vi "Run.vi"(8 "error in (no error)":errorcluster caption="entrée d'erreur (pas d'erreur)", 9 "y_score":string[][](array[string]), 10 "y_true":string[][](array[string]), 11 "Roc_Curve.lvclass":refnum<class "Roc_Curve.lvclass">) -> (0 "error out":errorcluster caption="sortie d'erreur", 2 "Data":T1, 3 "Roc_Curve.lvclass":refnum<class "Roc_Curve.lvclass">)   [LabVIEW 2020, in "Roc_Curve.lvclass"]
doc: "Returns :\n\n- fpr : array, shape = [>2]\nIncreasing false positive rates such that element i is the false positive rate of predictions with score >= thresholds[i].\n\n- tpr : array, shape = [>2]\nIncreasing true positive rates such that element i is the true positive rate of predictions with score >= thresholds[i].\n\n- thresholds : array, shape = [n_thresholds]\nDecreasing thresholds on the decision function used to compute fpr and tpr. thresholds[0] represents no instances being predicted and is arbitrarily set to max(y_score) + 1."
uses:
  Roc_Curve.lvclass
  Roc_Curve.lvclass/Roc_Curve.ctl
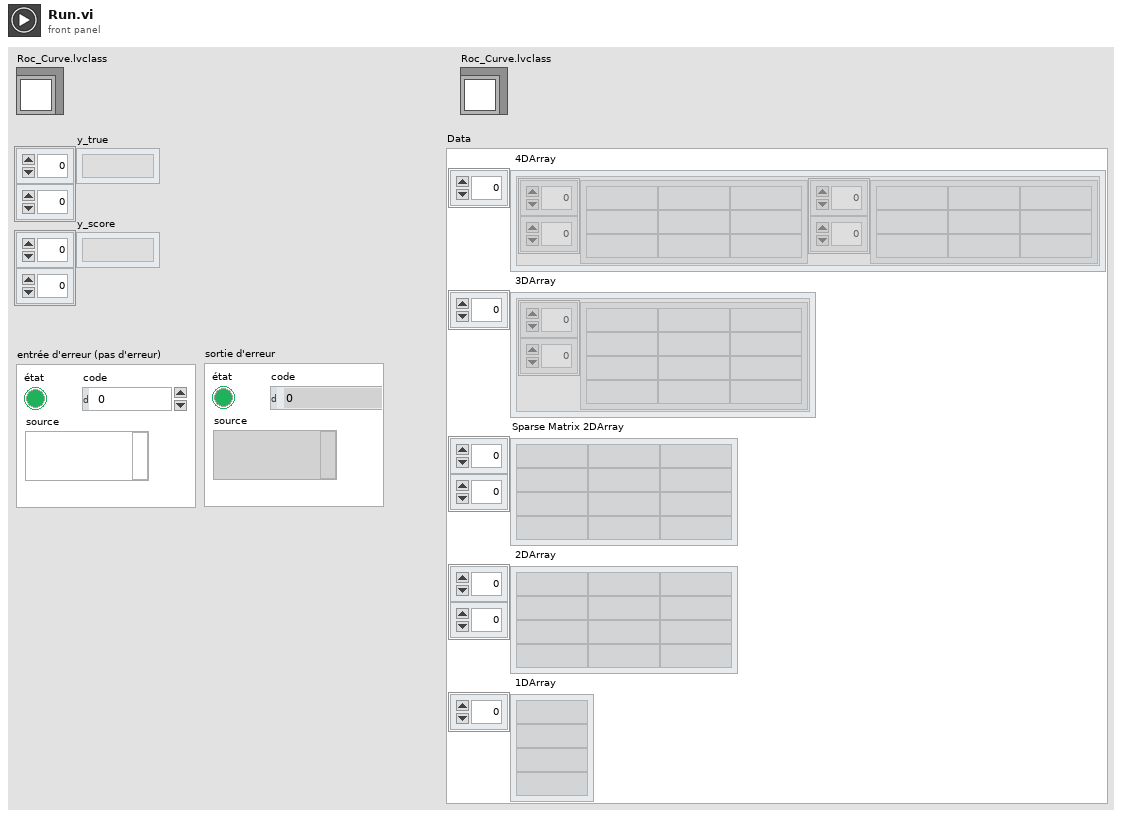
[diagram p1: front panel]
types:
  T1 = cluster{" 4DArray":cluster{"1":string[][], "2":string[][]}[], " 3DArray":cluster{"Tableau":string[][]}[], "Sparse Matrix 2DArray":string[][], " 2DArray":string[][], " 1DArray":string[]}
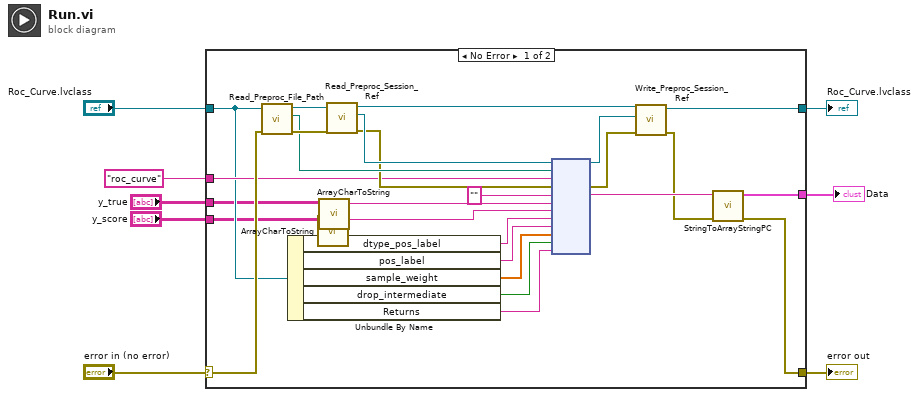
[diagram p0: block diagram]
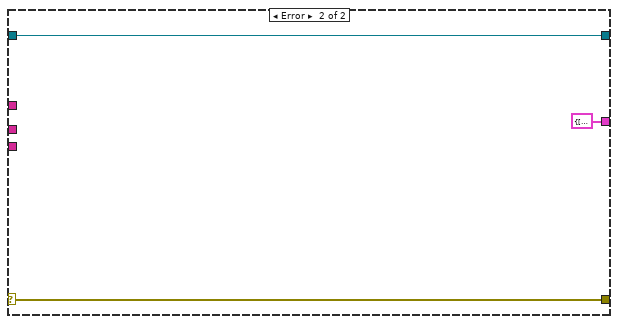
[diagram p2: hidden frame]
diagram:
  n1 = case shown="No Error" "error in (no error)" {
    selector: "error in (no error)" -> [w25 w37]
    tunnel: [w10 w37] -> w7
    tunnel: [w13 w36] -> w5
    tunnel: "Roc_Curve.lvclass" -> [w23 w36]
    tunnel: "roc_curve" -> [w24 _]
    tunnel: "y_true" -> [w17 _]
    tunnel: "y_score" -> [w16 _]
    tunnel: [w9 T1 {" 4DArray"=[], " 3DArray"=[], "Sparse Matrix 2DArray"=[], " 2DArray"=[], " 1DArray"=[]} ("Data")] -> w1
    frame No Error {
      n2 = call-dynamic "Read_Preproc_File_Path.vi"("error in (no error)"=w25, "Python in"=w23) -> ("error out"=w33:errorcluster, "File_Path"=w32:path, "Python out"=w34:refnum<class "Roc_Curve.lvclass">)  [unwired: 7 in]
      n3 = Unbundle By Name(w23) -> ("dtype_pos_label"=w22:string, "pos_label"=w21:string, "sample_weight"=w20:dbl[], "drop_intermediate"=w19:bool, "Returns"=w18:string)
      n4 = call "ArrayCharToString.vi"("TAB"=w16) -> ("Instruction"=w14:string)  [unwired: 10 in]
      n5 = call "ArrayCharToString.vi"("TAB"=w17) -> ("Instruction"=w15:string)  [unwired: 10 in]
      n6 = call-dynamic "Read_Preproc_Session_Ref.vi"("error in (no error)"=w33, "Python in"=w34) -> ("error out"=w30:errorcluster, "Session_ref"=w31:refnum<k35>, "Python out"=w29:refnum<class "Roc_Curve.lvclass">)  [unwired: 7 in]
      n7 = node(w31, w32, w24, w30, "", w15, w14, w22, w21, w20, w19, w18) -> (w27:refnum<k35>, w28:errorcluster, w12:string)  [unwired: 7 in, 2 out]
      n8 = call-dynamic "Write_Preproc_Session_Ref.vi"("error in (no error)"=w28, "Session_ref"=w27, "Python in"=w29) -> ("error out"=w11:errorcluster, "Python out"=w13:refnum<class "Roc_Curve.lvclass">)  [unwired: 7 in]
      n9 = call "StringToArrayStringPC.vi"("sortie d'erreur"=w11, "Return value"=w12) -> ("sortie d'erreur"=w10:errorcluster, "Data"=w9:T1)  [unwired: 8 in]
    }
    frame Error {
    }
  }
  "error out" <- w7
  "Roc_Curve.lvclass" <- w5
  "Data" <- w1
